vi "uService GUI.vi"(8 "error in (no error)":errorcluster, 11 "Monkey in":refnum<class "Monkey.lvclass">) -> (3 "Monkey out":refnum<class "Monkey.lvclass">)   [LabVIEW 2020, in "Monkey.lvlib" / "Monkey.lvclass"]
uses:
  Monkey.lvclass
  C:/Users/marco/Documents/GitHub_Lab/TALOS/talos/Father of all uServices/Father of all uServices/Father of all uServices.lvclass
  Run Utilities/Schedule/Array of Runs - GUI.ctl
  Run Utilities/Cell/Cell - GUI.ctl
  Run Utilities/Run Instance/Run Instance - GUI.ctl
  Ancestor/Ancestor/Ancestor.lvclass/Ancestor.ctl
  Support VIs/Substitute Error.vi
  Support VIs/Generate Error.vi
  FGV/Error Memory/Get Error Description.vi
  Support VIs/Get PC name.vi
  Ancestor/Ancestor/Read ID.vi
  Support VIs/Get Class Name.vi
  FGV/Error Memory/Error Memory Core.vi
  <vilib>/AdvancedString/Delimited String to 1D String Array.vi
  Support VIs/Circus Root Path.vi
  FGV/Error Memory/Error Crt Lvl checker.vi
  FGV/Error Memory/Error Memory Core.vi/40c8088d-b597-4017-91af-faa98e00292e.vi
  FGV/Error Memory/Error Memory Core.vi/d4a3ab98-063c-4e44-b43d-fbdcfe6c2be2.vi
  Father of all uServices/Father of all uServices/Father of all uServices.lvclass
  C:/Users/marco/Documents/GitHub_Lab/TALOS/builds/Actor Framework PPL/Actor Framework.lvlibp/1abvi3w/vi.lib/ActorFramework/Actor/Actor.lvclass
  builds/Actor Framework PPL/Actor Framework.lvlibp/1abvi3w/vi.lib/ActorFramework/Actor/Read Self Enqueuer.vi
  builds/Actor Framework PPL/Actor Framework.lvlibp/1abvi3w/vi.lib/ActorFramework/Stop Msg/Send Normal Stop.vi
  Support VIs/Global Memory.vi
  <vilib>/Utility/LVClass/Get LV Class Name.vi
  Support VIs/Is in Packed Library.vi
  Support VIs/TALOS Root path.vi
  Support VIs/Read CSV worksheet.vi
  Support VIs/Global Constants.vi
  <vilib>/Utility/error.llb/General Error Handler.vi
  Support VIs/Error Log.vi
  Ancestor/Ancestor/Ancestor.lvclass
  <vilib>/Comparison/Equal/Equal Functor/Equal Functor.lvclass
  Run Utilities/Run Instance/Run Instance.lvclass
  Run Utilities/Schedule/Schedule.lvclass
  Run Utilities/Cell/Schedule Cell.lvclass
panel:
  in  "Skip schedule":bool
  out "Stopped":bool
  out "Paused":bool
  in  "Monkey Picture":picture
  out "Error Criticality":u8 max=4
  out "uS ID":string
  out "Synchronised":bool
  out "Continuous":bool
  out "Current RUN":T1
  out "ETA":string
  out "Scripts left":dbl
  out "Skipped RUNs":T2 {"Number of cycles" min=1}
  out "Report from previous RUNs":string
  out "Current Action":string
  out "RUNs Schedule":T2 {"Number of cycles" min=1}
  in  "stop Monkey":bool
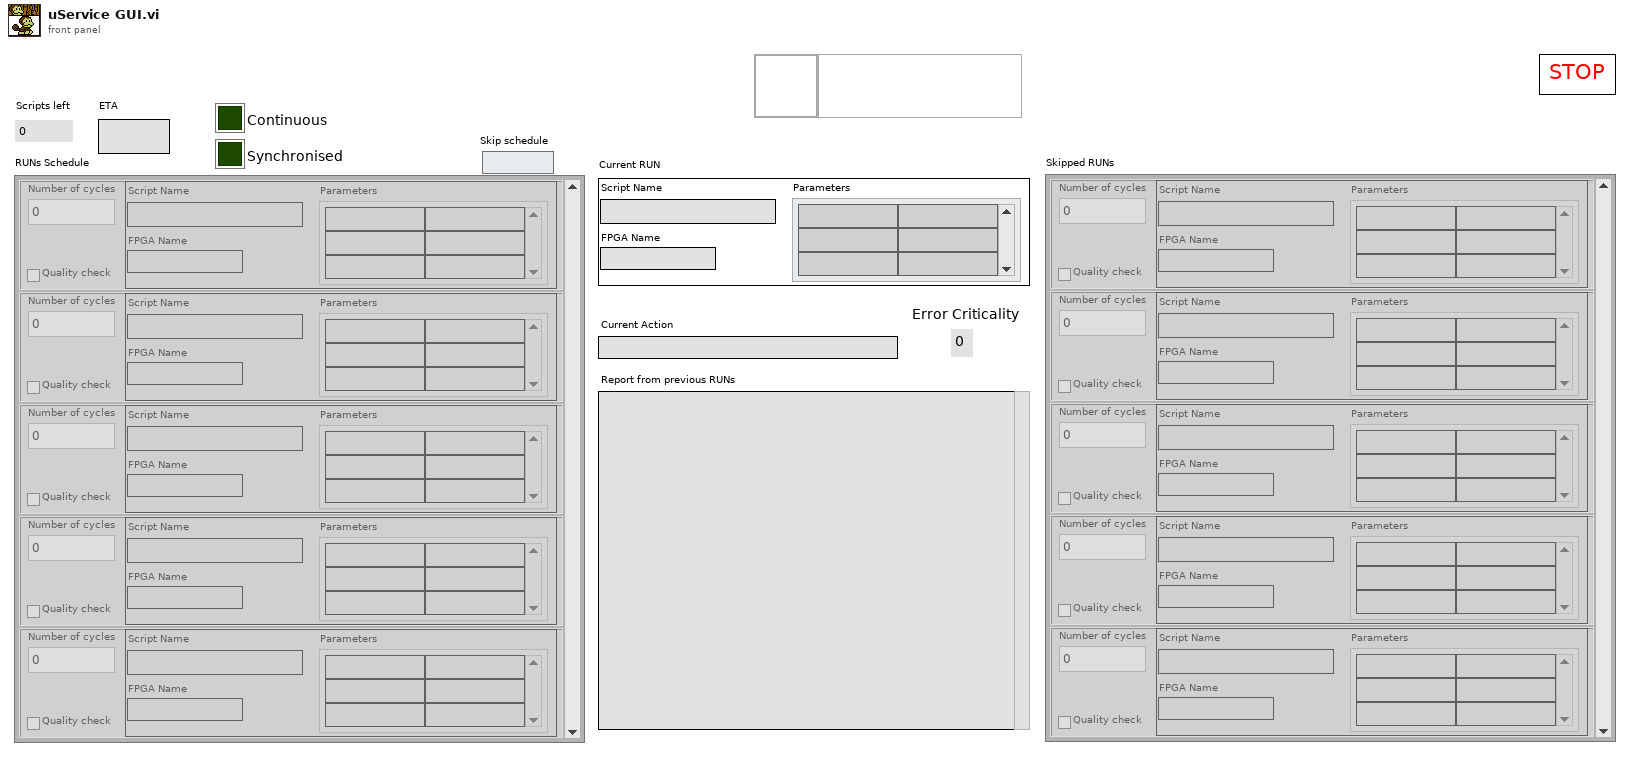
[diagram p1: front panel]
types:
  T1 = typedef "TALOS.lvlib/Run Utilities.lvlib/Run Instance.lvclass/Run Instance - GUI.ctl" = cluster{"Script Name":string, "Parameters":string[][], "FPGA Name":string}
  T2 = typedef "TALOS.lvlib/Run Utilities.lvlib/Schedule.lvclass/Array of Runs - GUI.ctl" = T3[]
  T3 = typedef "TALOS.lvlib/Run Utilities.lvlib/Schedule Cell.lvclass/Cell - GUI.ctl" = cluster{"Background Color":u32, "Number of cycles":u32, "Single RUN":T1, "Quality check":bool, "Cell Type":string}
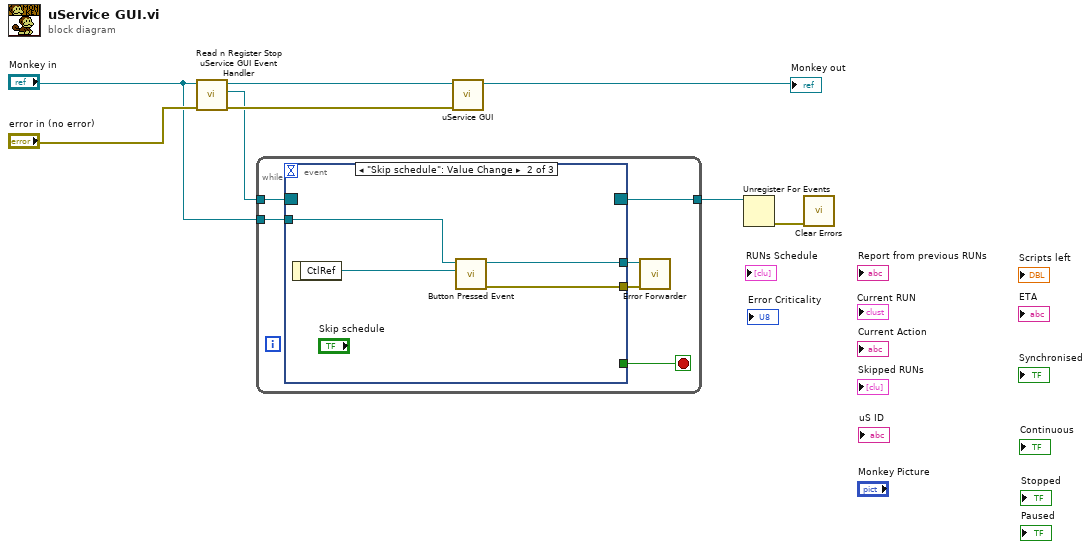
[diagram p0: block diagram]
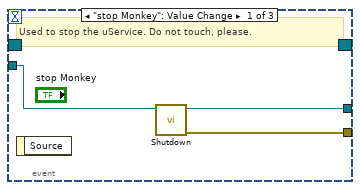
[diagram p2: hidden frame]
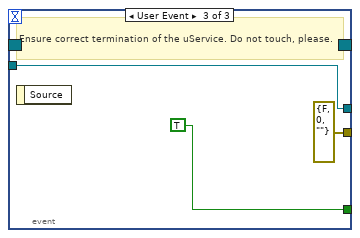
[diagram p3: hidden frame]
diagram:
  n1 = call-dynamic "Read n Register Stop uService GUI Event Handler .vi"("error in (no error)"="error in (no error)", "uService Template in"="Monkey in") -> ("error out"=w6:errorcluster, "Stop uService GUI Event Ref"=w5:refnum<event-registration>, "uService Template out"=w7:refnum<class "Monkey.lvclass">)  [unwired: 7 in]
  n2 = while {
    tunnel: [w14] -> w8
    tunnel: w5 -> [w12]
    tunnel: "Monkey in" -> [w11]
    stop <- w13 stop-if-true
    n3 = event shown="[1] \"Skip schedule\": Value Change" {
      selector: w12 -> [_ _ _]
      dyn-events: [_ _ _] -> w14
      timeout: _ -> [_ _ _]
      tunnel: [_ _ TRUE] -> w13
      tunnel: w11 -> [w17 w21 w23]
      tunnel: [w16 w19 w23] -> w10
      tunnel: [w15 w18 errorcluster {"status"=FALSE, "code"=0, "source"=""} ("error out")] -> w9
      event "stop Monkey": Value Change {
        # "Used to stop the uService. Do not touch, please."
        n4 = event-data() -> ()  [unwired: 1 in, 1 out]
        n5 = call "Shutdown.vi"("Father of all uServices in"=w17) -> ("error out"=w15:errorcluster, "Father of all uServices out"=w16:refnum<class "Monkey.lvclass">)  [unwired: 9 in]
      }
      event "Skip schedule": Value Change {
        n6 = event-data() -> ("CtlRef"=w20:refnum<vi>)  [unwired: 1 in]
        n7 = call-dynamic "Button Pressed Event.vi"("CtlRef"=w20, "uService Template in"=w21) -> ("error out"=w18:errorcluster, "uService Template out"=w19:refnum<class "Monkey.lvclass">)  [unwired: 8 in]
      }
      event User Event {
        # "Ensure correct termination of the uService. Do not touch, please."
        n8 = event-data() -> ()  [unwired: 1 in, 1 out]
      }
    }
    n9 = call "Error Forwarder.vi"("error in (no error)"=w9, "Father of all uServices in"=w10) -> ()  [unwired: 10 in]
  }
  n10 = call-parent "uService GUI.vi"("error in (no error)"=w6, "uService Template in"=w7) -> ("uService Template out"=→"Monkey out":refnum<class "Monkey.lvclass">)  [unwired: 9 in]
  n11 = Unregister For Events(event registration refnum=w8) -> (error out=w1:errorcluster)  [unwired: 1 in]
  n12 = call <vilib>:"Clear Errors.vi"("error in (no error)"=w1) -> ()  [unwired: 5 in, 2 out]
